vi "Numeric_bins.vi"(0 "Values":dbl[](array[numeric]) format="%.4f", 1 "Tolerance":dbl=0.02 format="%.3f") -> (2 "Bin Centres":dbl[](array[numeric]) format="%.4f", 3 "No of points in bins":i32[](array[numeric]), 4 "Bin Index":i32[](array[numeric]))   [LabVIEW 2020]
panel:
  out "Offset":dbl
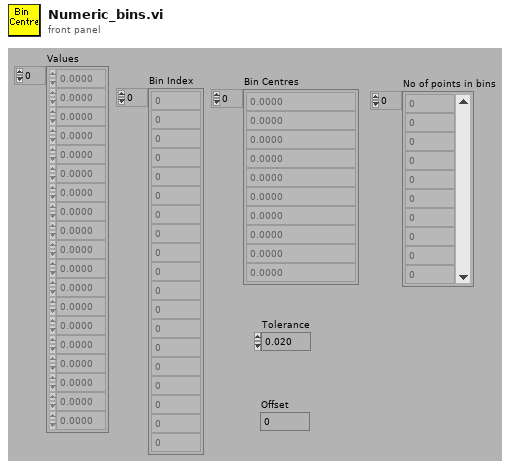
[diagram p1: front panel]
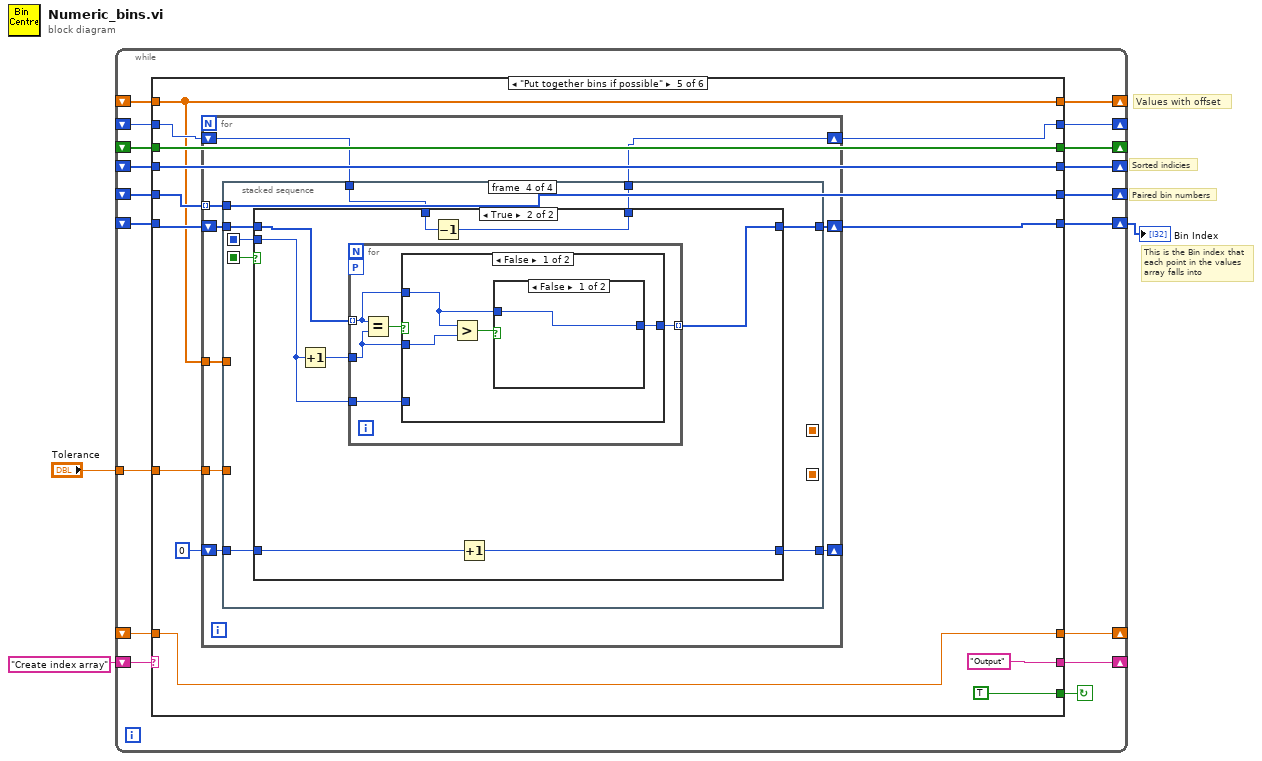
[diagram p0: block diagram]
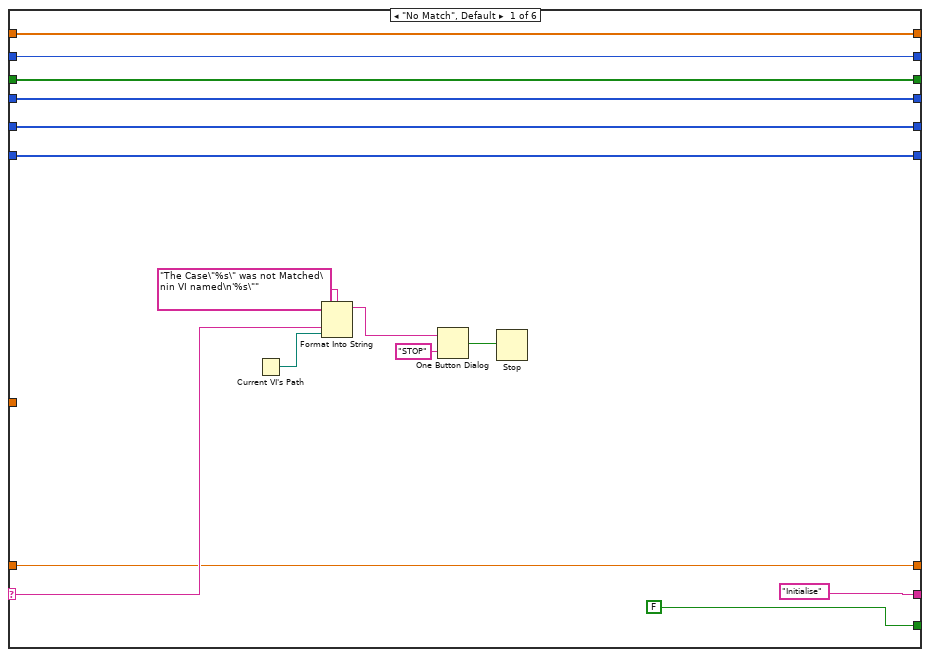
[diagram p2: hidden frame]
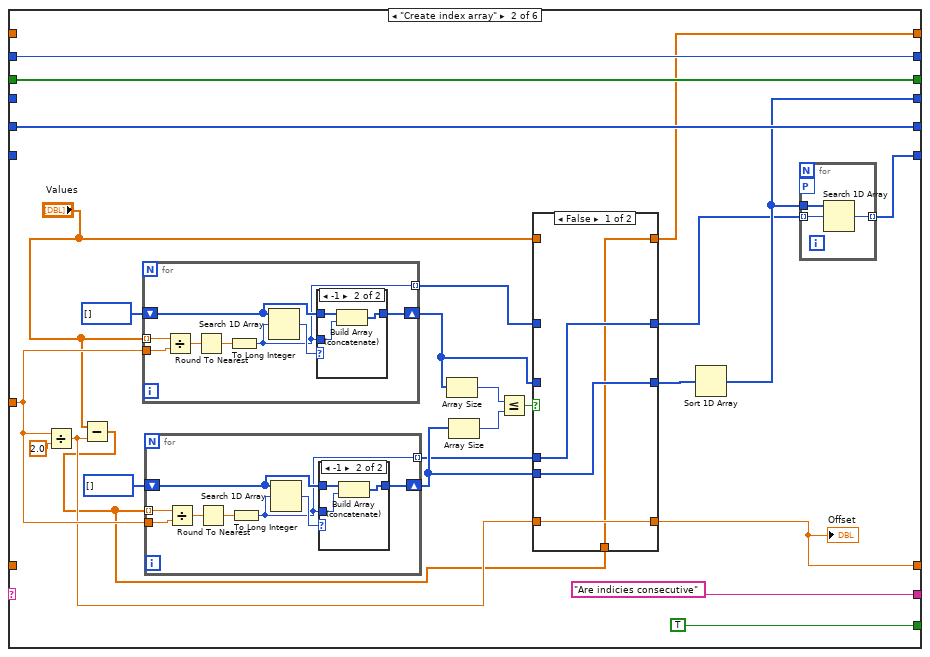
[diagram p3: hidden frame]
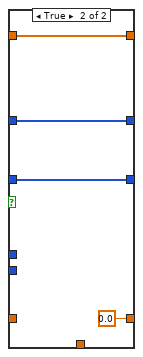
[diagram p4: hidden frame]
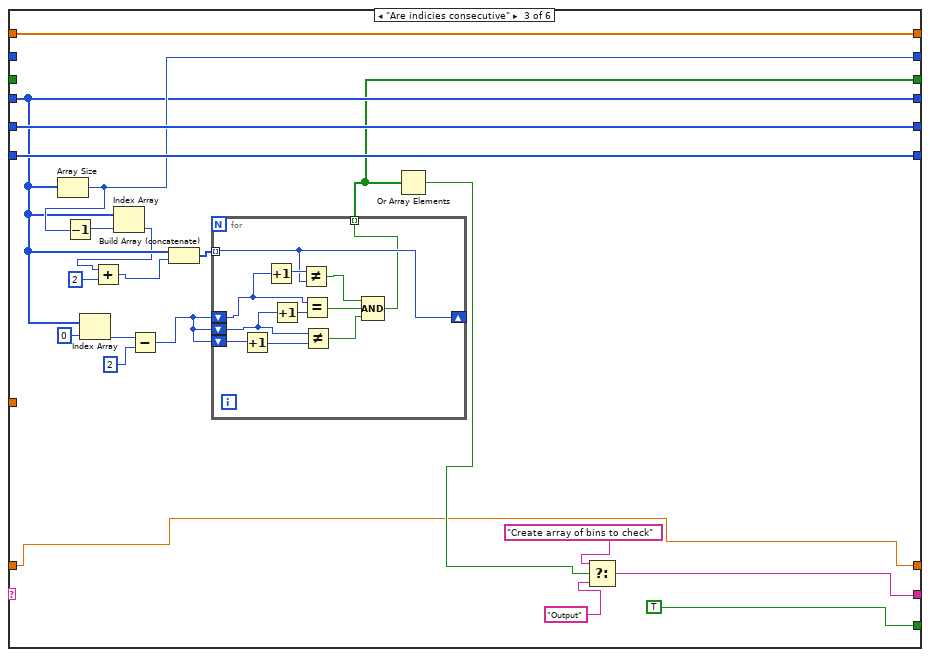
[diagram p7: hidden frame]
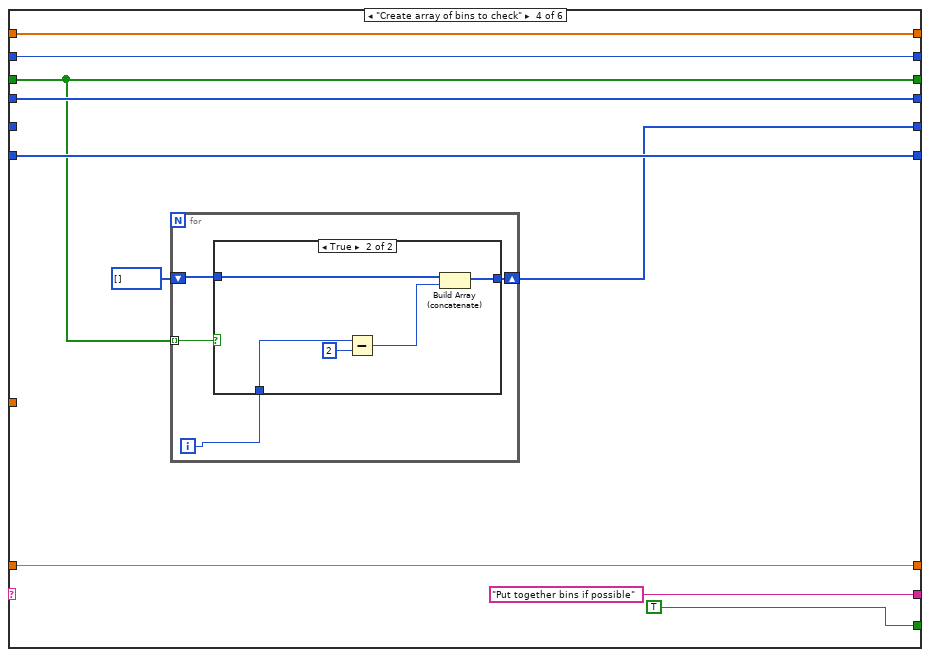
[diagram p8: hidden frame]
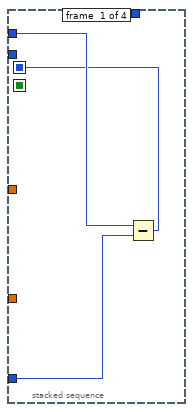
[diagram p10: hidden frame]
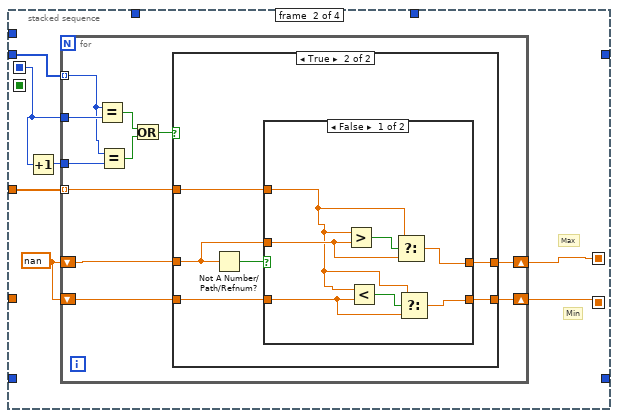
[diagram p11: hidden frame]
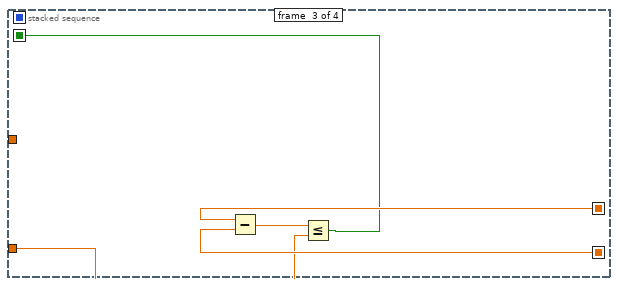
[diagram p14: hidden frame]
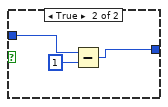
[diagram p16: hidden frame]
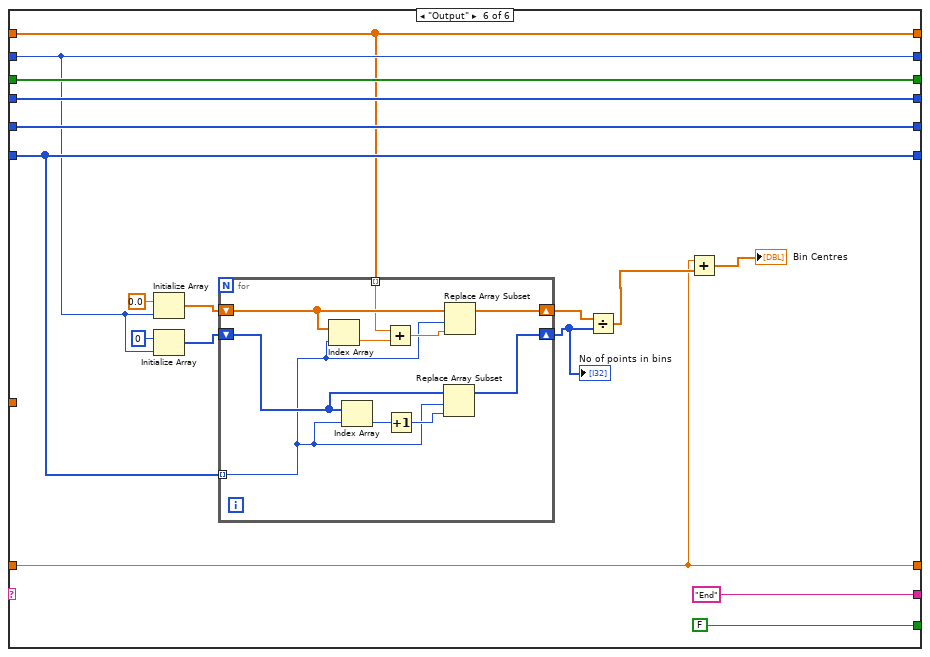
[diagram p18: hidden frame]
diagram:
  # "Values with offset"
  # "Paired bin numbers"
  # "This is the Bin index that\neach point in the values\narray falls into"
  # "Sorted indicies"
  n1 = while {
    shift-left: "Create index array" -> [w19]
    shift-right: [w20] -> _
    shift-right: [w18] -> _
    shift-left: _ -> [w14]
    shift-right: [w17] -> _
    shift-left: _ -> [w15]
    tunnel: "Tolerance" -> [w16]
    shift-right: [w13] -> _
    shift-left: _ -> [w11]
    shift-right: [w12] -> w2
    shift-left: _ -> [w10]
    shift-right: [w9] -> _
    shift-left: _ -> [w8]
    shift-right: [w7] -> _
    shift-left: _ -> [w6]
    shift-right: [w5] -> _
    shift-left: _ -> [w4]
    stop <- w21 continue-if-true
    n2 = case shown="\"Put together bins if possible\"" w19 {
      selector: w19 -> [w24 _ _ _ _ _]
      tunnel: [FALSE TRUE TRUE TRUE TRUE FALSE] -> w21
      tunnel: ["Initialise" "Are indicies consecutive" w111 "Put together bins if possible" "Output" "End"] -> w20
      tunnel: [w28 w58 w105 w136 w160 w256] -> w18
      tunnel: [w29 w56 w100 w134 w159 w257] -> w17
      tunnel: w16 -> [_ w52 _ _ w157 _]
      tunnel: w15 -> [w29 w56 _ w134 w159 w257]
      tunnel: w14 -> [w28 _ w105 w136 w160 w256]
      tunnel: [w27 w59 w116 w131 w158 w252] -> w13
      tunnel: [w26 w57 w115 w137 w155 w253] -> w12
      tunnel: w11 -> [w27 w59 w116 _ w158 w252]
      tunnel: w10 -> [w26 _ w115 w137 w156 w253]
      tunnel: [w25 w55 w107 w133 w153 w251] -> w9
      tunnel: w8 -> [w25 w55 _ w133 w152 w251]
      tunnel: [w23 w41 w98 w130 w150 w247] -> w7
      tunnel: w6 -> [w23 _ w98 w130 w150 w247]
      tunnel: [w22 w39 w97 w129 w149 w246] -> w5
      tunnel: w4 -> [w22 _ w97 w129 w149 w246]
      frame "No Match", Default {
        n3 = Current VI's Path() -> (path=w31:path)
        n4 = Format Into String(format string="The Case\"%s\" was not Matched\nin VI named\n'%s\"" ("Format String"), w24, w31) -> (resulting string=w34:string)  [unwired: 2 in, 1 out]
        n5 = One Button Dialog(message=w34, button name ("OK")="STOP") -> (true=w32:bool)
        n6 = Stop(stop? (T)=w32) -> ()
      }
      frame "Create index array" {
        n7 = Divide(x=w52, y=2.0) -> (x/y=w40:dbl)
        n8 = Subtract(x="Values", y=w40) -> (x-y=w38:dbl[])
        n9 = for {
          shift-right: [w91] -> w46
          shift-left: i32[] [] -> [w90]
          tunnel: "Values" -> [w88] mode=indexing
          tunnel: w52 -> [w87]
          tunnel: [w85] -> w44 mode=indexing
          n10 = Divide(x=w88, y=w87) -> (x/y=w86:dbl)
          n11 = Round To Nearest(number=w86) -> (nearest integer value=w89:dbl)
          n12 = To Long Integer(number=w89) -> (32bit integer=w85:i32)
          n13 = Search 1D Array(1D array=w90, element=w85) -> (index of element=w92:i32)  [unwired: 1 in]
          n14 = case shown="-1" w92 {
            tunnel: w90 -> [w93 w96]
            tunnel: w85 -> [_ w94]
            tunnel: [w93 w95] -> w91
            frame 0, Default {
            }
            frame -1 {
              n15 = Build Array (concatenate)(w96, w94) -> (w95:i32[])
            }
          }
        }
        n16 = for {
          shift-right: [w76] -> w45
          shift-left: i32[] [] -> [w75]
          tunnel: w38 -> [w73] mode=indexing
          tunnel: w52 -> [w72]
          tunnel: [w70] -> w42 mode=indexing
          n17 = Divide(x=w73, y=w72) -> (x/y=w71:dbl)
          n18 = Round To Nearest(number=w71) -> (nearest integer value=w74:dbl)
          n19 = To Long Integer(number=w74) -> (32bit integer=w70:i32)
          n20 = Search 1D Array(1D array=w75, element=w70) -> (index of element=w77:i32)  [unwired: 1 in]
          n21 = case shown="-1" w77 {
            tunnel: w75 -> [w78 w81]
            tunnel: w70 -> [_ w79]
            tunnel: [w78 w80] -> w76
            frame 0, Default {
            }
            frame -1 {
              n22 = Build Array (concatenate)(w81, w79) -> (w80:i32[])
            }
          }
        }
        n23 = Array Size(array=w46) -> (size(s)=w50:i32)
        n24 = Array Size(array=w45) -> (size(s)=w49:i32)
        n25 = Less Or Equal?(x=w50, y=w49) -> (x <= y?=w48:bool)
        n26 = case shown="False" w48 {
          tunnel: [w65 w69] -> w47
          tunnel: w46 -> [_ w69]
          tunnel: w45 -> [w65 _]
          tunnel: [w64 w68] -> w43
          tunnel: w44 -> [_ w68]
          tunnel: w42 -> [w64 _]
          tunnel: [w63 0.0] -> w41
          tunnel: w40 -> [w63 _]
          tunnel: [w62 w66] -> w39
          tunnel: "Values" -> [_ w66]
          tunnel: w38 -> [w62 _]
          frame False {
          }
          frame True {
          }
        }
        "Offset" <- w41
        n27 = Sort 1D Array(array=w47) -> (sorted array=w58:i32[])
        n28 = for {
          tunnel: w58 -> [w84]
          tunnel: w43 -> [w83] mode=indexing
          tunnel: [w82] -> w57 mode=indexing
          workers-P: _ -> [_]
          n29 = Search 1D Array(1D array=w84, element=w83) -> (index of element=w82:i32)  [unwired: 1 out]
        }
      }
      frame "Are indicies consecutive" {
        n30 = Array Size(array=w105) -> (size(s)=w107:i32)
        n31 = Decrement(x=w107) -> (x-1=w106:i32)
        n32 = Index Array(array=w105, index=0) -> (element=w113:i32)
        n33 = Index Array(array=w105, index=w106) -> (element=w104:i32)
        n34 = Add(x=w104, y=2) -> (x+y=w102:i32)
        n35 = Subtract(x=w113, y=2) -> (x-y=w108:i32)
        n36 = Build Array (concatenate)(w105, w102) -> (w101:i32[])
        n37 = for {
          shift-right: [w122] -> _
          shift-left: w108 -> [w124]
          tunnel: w101 -> [w122] mode=indexing
          tunnel: [w118] -> w100 mode=indexing
          shift-left: w108 -> [w126]
          shift-left: w108 -> [w128]
          n38 = Increment(x=w128) -> (x+1=w127:i32)
          n39 = Increment(x=w124) -> (x+1=w123:i32)
          n40 = Increment(x=w126) -> (x+1=w125:i32)
          n41 = Not Equal?(x=w123, y=w122) -> (x != y?=w121:bool)
          n42 = Equal?(x=w124, y=w125) -> (x = y?=w120:bool)
          n43 = Not Equal?(x=w126, y=w127) -> (x != y?=w119:bool)
          n44 = Compound Arithmetic op=AND(w121, w120, w119) -> (w118:bool)
        }
        n45 = Or Array Elements(Boolean array=w100) -> (logical OR=w99:bool)
        n46 = Select(t="Create array of bins to check", s=w99, f="Output") -> (s? t:f=w111:string)
      }
      frame "Create array of bins to check" {
        n47 = for {
          tunnel: w134 -> [w142] mode=indexing
          shift-right: [w139] -> w131
          shift-left: i32[] [] -> [w140]
          i -> [w141]
          n48 = case shown="True" w142 {
            tunnel: w141 -> [_ w148]
            tunnel: w140 -> [w143 w146]
            tunnel: [w143 w144] -> w139
            frame False {
            }
            frame True {
              n49 = Subtract(x=w148, y=2) -> (x-y=w145:i32)
              n50 = Build Array (concatenate)(w146, w145) -> (w144:i32[])
            }
          }
        }
      }
      frame "Put together bins if possible" {
        n51 = for {
          tunnel: w158 -> [w170] mode=indexing
          tunnel: w149 -> [w169]
          tunnel: w157 -> [w168]
          shift-right: [w167] -> w155
          shift-left: w156 -> [w166]
          shift-right: [w164] -> w153
          shift-left: w152 -> [w165]
          shift-right: [w163] -> _
          shift-left: 0 -> [w162]
          n52 = stacked-sequence {
            seq-local: [_ w178 _ _] -> [_ _ w212 _]
            seq-local: [_ w177 _ _] -> [_ _ w211 _]
            seq-local: [_ _ w208 _] -> [_ _ _ w220]
            seq-local: [w171 _ _ _] -> [_ w174 _ w213]
            tunnel: w170 -> [w173 _ _ _]
            tunnel: w169 -> [_ w179 _ _]
            tunnel: w168 -> [_ _ w209 _]
            tunnel: [_ _ _ w219] -> w167
            tunnel: w166 -> [_ w175 _ w218]
            tunnel: w165 -> [_ _ _ w217]
            tunnel: [_ _ _ w216] -> w164
            tunnel: [_ _ _ w215] -> w163
            tunnel: w162 -> [w172 _ _ w214]
            frame #0 {
              n53 = Subtract(x=w173, y=w172) -> (x-y=w171:i32)
            }
            frame #1 {
              w180 = nan
              # "Min"
              # "Max"
              n54 = Increment(x=w174) -> (x+1=w176:i32)
              n55 = for {
                tunnel: w174 -> [w191]
                shift-right: [w185] -> w178
                shift-left: w180 -> [w187]
                shift-right: [w184] -> w177
                shift-left: w180 -> [w183]
                tunnel: w179 -> [w186] mode=indexing
                tunnel: w176 -> [w182]
                tunnel: w175 -> [w181] mode=indexing
                n56 = Equal?(x=w181, y=w191) -> (x = y?=w189:bool)
                n57 = Equal?(x=w181, y=w182) -> (x = y?=w190:bool)
                n58 = Or(x=w189, y=w190) -> (x .or. y?=w188:bool)
                n59 = case shown="True" w188 {
                  tunnel: w187 -> [w193 w195]
                  tunnel: w186 -> [_ w198]
                  tunnel: [w193 w197] -> w185
                  tunnel: [w192 w196] -> w184
                  tunnel: w183 -> [w192 w194]
                  frame False {
                  }
                  frame True {
                    n60 = Not A Number/Path/Refnum?(number/path/refnum=w195) -> (NaN/Path/Refnum?=w199:bool)
                    n61 = case shown="False" w199 {
                      tunnel: w198 -> [w202 w207]
                      tunnel: [w204 w207] -> w197
                      tunnel: [w200 w207] -> w196
                      tunnel: w195 -> [w205 _]
                      tunnel: w194 -> [w201 _]
                      frame False {
                        n62 = Greater?(x=w202, y=w205) -> (0:w206:bool)
                        n63 = Less?(x=w202, y=w201) -> (x < y?=w203:bool)
                        n64 = Select(t=w202, s=w206, f=w205) -> (s? t:f=w204:dbl)
                        n65 = Select(t=w202, s=w203, f=w201) -> (s? t:f=w200:dbl)
                      }
                      frame True {
                      }
                    }
                  }
                }
              }
            }
            frame #2 {
              n66 = Subtract(x=w212, y=w211) -> (x-y=w210:dbl)
              n67 = Less Or Equal?(x=w210, y=w209) -> (x <= y?=w208:bool)
            }
            frame #3 {
              n68 = case shown="True" w220 {
                tunnel: [w223 w229] -> w219
                tunnel: w218 -> [w223 w230]
                tunnel: w217 -> [w222 w228]
                tunnel: [w222 w227] -> w216
                tunnel: [w221 w224] -> w215
                tunnel: w214 -> [w221 w225]
                tunnel: w213 -> [_ w226]
                frame False {
                }
                frame True {
                  n69 = Increment(x=w226) -> (x+1=w231:i32)
                  n70 = for {
                    tunnel: w231 -> [w232]
                    tunnel: w230 -> [w233] mode=indexing
                    tunnel: [w235] -> w229 mode=indexing
                    tunnel: w226 -> [w234]
                    workers-P: _ -> [_]
                    n71 = Equal?(x=w233, y=w232) -> (x = y?=w236:bool)
                    n72 = case shown="False" w236 {
                      tunnel: [w237 w245] -> w235
                      tunnel: w234 -> [_ w245]
                      tunnel: w233 -> [w238 _]
                      tunnel: w232 -> [w240 _]
                      frame False {
                        n73 = Greater?(x=w238, y=w240) -> (0:w239:bool)
                        n74 = case shown="False" w239 {
                          tunnel: w238 -> [w241 w244]
                          tunnel: [w241 w242] -> w237
                          frame False {
                          }
                          frame True {
                            n75 = Subtract(x=w244, y=1) -> (x-y=w242:i32)
                          }
                        }
                      }
                      frame True {
                      }
                    }
                  }
                  n76 = Decrement(x=w228) -> (x-1=w227:i32)
                  n77 = Increment(x=w225) -> (x+1=w224:i32)
                }
              }
            }
          }
        }
      }
      frame "Output" {
        n78 = Initialize Array(0.0 ("element"), w251) -> (w259:dbl[])
        n79 = Initialize Array(0 ("element"), w251) -> (w261:i32[])
        n80 = for {
          shift-right: [w271] -> w262
          shift-left: w259 -> [w272]
          shift-right: [w270] -> w250
          shift-left: w261 -> [w269]
          tunnel: w246 -> [w264] mode=indexing
          tunnel: w253 -> [w263] mode=indexing
          n81 = Index Array(array=w272, index=w263) -> (element=w266:dbl)
          n82 = Index Array(array=w269, index=w263) -> (element=w268:i32)
          n83 = Add(x=w264, y=w266) -> (x+y=w265:dbl)
          n84 = Increment(x=w268) -> (x+1=w267:i32)
          n85 = Replace Array Subset(array=w269, new element=w267, index=w263) -> (w270:i32[])
          n86 = Replace Array Subset(array=w272, new element=w265, index=w263) -> (w271:dbl[])
        }
        "No of points in bins" <- w250
        n87 = Divide(x=w262, y=w250) -> (x/y=w249:dbl[])
        n88 = Add(x=w247, y=w249) -> (x+y=→"Bin Centres":dbl[])
      }
    }
  }
  "Bin Index" <- w2
